vi "CheckShots2Ship.vi"(6 "IntensityArray_IN":u8[][](array[numeric]), 7 "SpaceshipPosition":T1, 11 "ShotArray_IN":T2[](array[typedef])) -> (3 "ShotArray_OUT":T2[](array[typedef]), 4 "IntensityArray_OUT":u8[][](array[numeric]), 5 "GameOver":bool)   [LabVIEW 2022 SP3]
uses:
  ShotCluster.ctl
  move_dir_ud.ctl
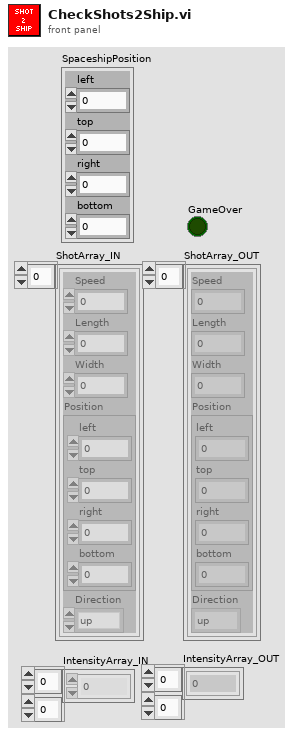
[diagram p1: front panel]
types:
  T1 = cluster{"left":i16, "top":i16, "right":i16, "bottom":i16}
  T2 = typedef "ShotCluster.ctl" = cluster{"Speed":u32, "Length":u32, "Width":u32, "Position":cluster{"left":i16, "top":i16, "right":i16, "bottom":i16}, "Direction":T3}
  T3 = typedef "move_dir_ud.ctl" = enum16{"up", "down"}
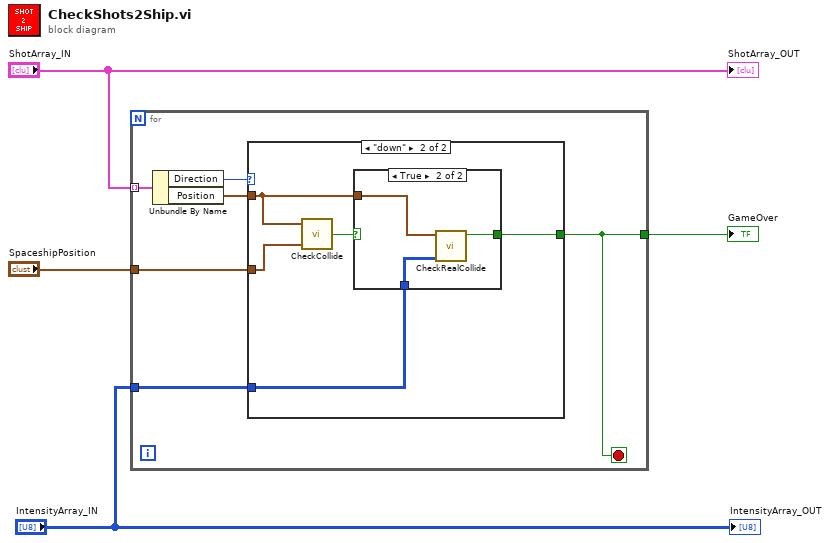
[diagram p0: block diagram]
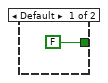
[diagram p2: hidden frame]
diagram:
  n1 = for {
    tunnel: "ShotArray_IN" -> [w10] mode=indexing
    tunnel: "SpaceshipPosition" -> [w8]
    tunnel: [w6] -> w2
    tunnel: "IntensityArray_IN" -> [w5]
    stop <- w6 stop-if-true
    n2 = Unbundle By Name(w10) -> ("Direction"=w9:T3, "Position"=w7:T1)
    n3 = case shown="\"down\"" w9 {
      tunnel: w8 -> [_ w16]
      tunnel: w7 -> [_ w12]
      tunnel: [FALSE ("Collide") w14] -> w6
      tunnel: w5 -> [_ w13]
      frame Default {
      }
      frame "down" {
        n4 = call "CheckCollide.vi"("Rectangle2"=w16, "Rectangle1"=w12) -> ("Collide"=w15:bool)  [unwired: 3 in]
        n5 = case shown="True" w15 {
          selector: w15 -> [w17 _]
          tunnel: [w17 w18] -> w14
          tunnel: w13 -> [_ w19]
          tunnel: w12 -> [_ w20]
          frame False {
          }
          frame True {
            n6 = call "CheckRealCollide.vi"("IntensityArray_IN"=w19, "ShotPosition"=w20) -> ("RealCollide?"=w18:bool)  [unwired: 9 in]
          }
        }
      }
    }
  }
  "GameOver" <- w2
  "ShotArray_OUT" <- "ShotArray_IN"
  "IntensityArray_OUT" <- "IntensityArray_IN"
